vi "Phase_unwrapping.vi"(10 "dt":dbl format="%#_13g", 11 "phase":dbl[](array[numeric])) -> (3 "phase difference":dbl[](array[numeric]))   [LabVIEW 2016]
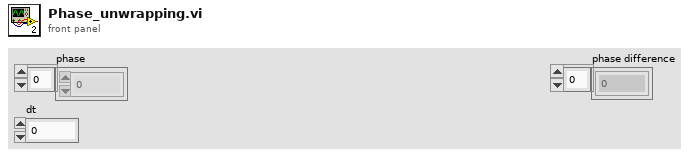
[diagram p1: front panel]
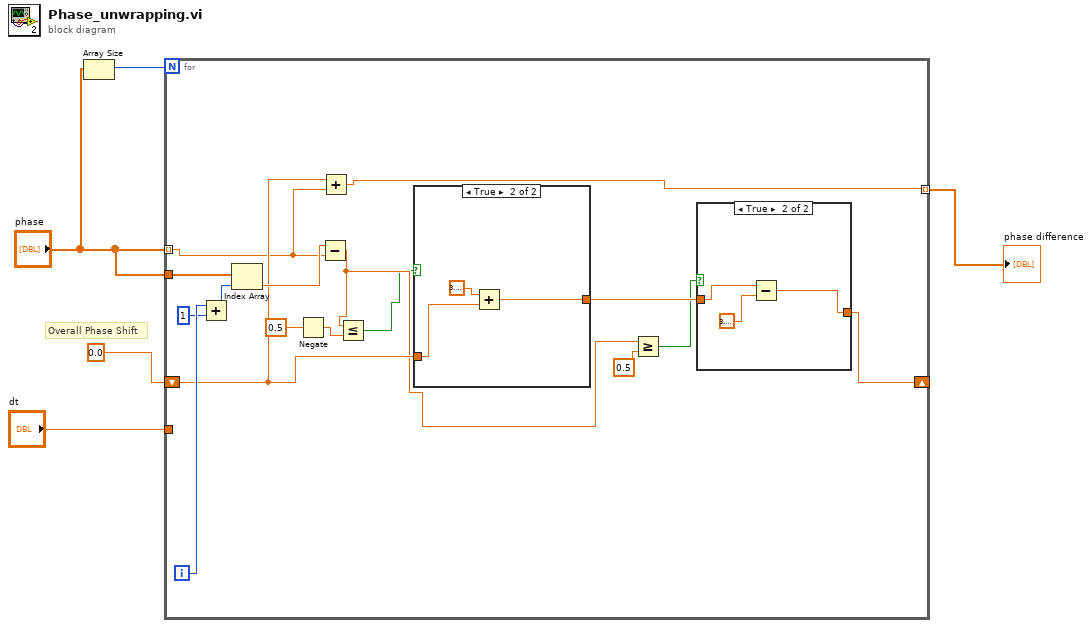
[diagram p0: block diagram]
diagram:
  # "Overall Phase Shift"
  n1 = Array Size(array="phase") -> (size(s)=w5:i32)
  n2 = for {
    N: w5 -> [_]
    tunnel: "phase" -> [w15] mode=indexing
    tunnel: "phase" -> [w21]
    tunnel: "dt" -> [_]
    shift-right: [w10] -> _
    shift-left: 0.0 -> [w16]
    tunnel: [w14] -> w1 mode=indexing
    i -> [w20]
    n3 = Add(x=w20, y=1) -> (x+y=w18:i32)
    n4 = Index Array(array=w21, index=w18) -> (element=w17:dbl)
    n5 = Negate(x=0.5) -> (-x=w8:dbl)
    n6 = Subtract(x=w17, y=w15) -> (x-y=w12:dbl)
    n7 = Add(x=w16, y=w15) -> (x+y=w14:dbl)
    n8 = Less Or Equal?(x=w12, y=w8) -> (x <= y?=w9:bool)
    n9 = case shown="True" w9 {
      tunnel: w16 -> [w26 w29]
      tunnel: [w26 w27] -> w13
      frame False {
      }
      frame True {
        n10 = Add(x=3.141592653589793, y=w29) -> (x+y=w27:dbl)
      }
    }
    n11 = Greater Or Equal?(x=w12, y=0.5) -> (x >= y?=w11:bool)
    n12 = case shown="True" w11 {
      tunnel: w13 -> [w22 w24]
      tunnel: [w22 w23] -> w10
      frame False {
      }
      frame True {
        n13 = Subtract(x=w24, y=3.141592653589793) -> (x-y=w23:dbl)
      }
    }
  }
  "phase difference" <- w1
